vi "FTW-XML-Query-ElementXML.vi"(0 "XML Node":refnum<k20>, 5 "XPath":string, 11 "error in":errorcluster) -> (4 "XML Node out":refnum<k20>, 6 "Node XML":string, 8 "Found?":bool, 15 "error out":errorcluster)   [LabVIEW 2012]
uses:
  Error/FTW-ERR-ThrowError.vi
  <resource>/objmgr/DOMUserDefRef.rc
panel:
  # "Inputs"
  # "Outputs"
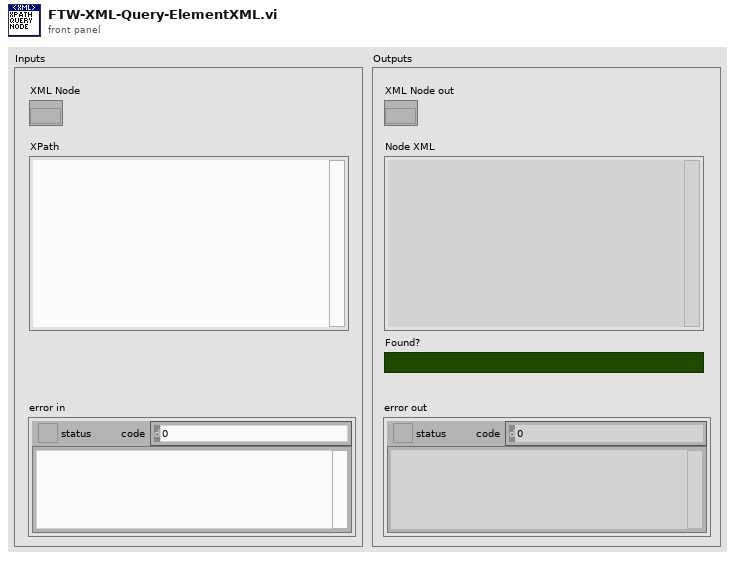
[diagram p1: front panel]
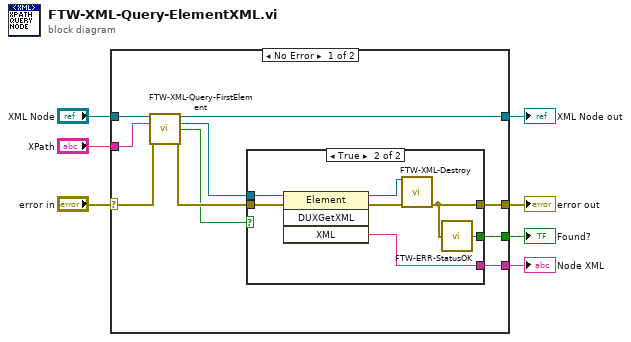
[diagram p0: block diagram]
diagram:
  n1 = case shown="No Error" "error in" {
    selector: "error in" -> [w10 w27]
    tunnel: [w17 w27] -> w7
    tunnel: "XML Node" -> [w14 w26]
    tunnel: [w13 w26] -> w4
    tunnel: "XPath" -> [w11 _]
    tunnel: [w16 _] -> w2
    tunnel: [w15 _] -> w1
    frame No Error {
      n2 = call "FTW-XML-Query-FirstElement.vi"("XML Node"=w14, "XPath Query"=w11, "error in"=w10) -> ("XML Node out"=w13:refnum<k20>, "First Matched Element"=w12:refnum<k20>, "Found?"=w8:bool, "error out"=w9:errorcluster)  [unwired: 8 in, 1 out]
      n3 = case shown="True" w8 {
        tunnel: w9 -> [w18 w25]
        tunnel: [w18 w19] -> w17
        tunnel: [_ w22] -> w16
        tunnel: w12 -> [_ w24]
        tunnel: [_ w23] -> w15
        frame False {
        }
        frame True {
          n4 = invoke class="Element" method="DUXGetXML"(reference=w24, error in=w25) -> (reference out=w21:refnum<k20>, error out=w20:errorcluster, "XML"=w22:string)  [unwired: 2 in, 1 out]
          n5 = call "FTW-XML-Destroy.vi"("XML Node"=w21, "error in"=w20) -> ("error out"=w19:errorcluster)  [unwired: 13 in]
          n6 = call "FTW-ERR-StatusOK.vi"("error to check"=w19) -> ("Status OK?"=w23:bool)
        }
      }
    }
    frame Error {
    }
  }
  "error out" <- w7
  "XML Node out" <- w4
  "Found?" <- w1
  "Node XML" <- w2
